vi "拉取dll文件.vi"(9 "添加的路径":path, 10 "MD5 message-digest":string="47126f942acc1a6f17c5325a05c10f2e", 11 "名称或相对路径":string="FreeMem.dll") -> (0 "error out":errorcluster caption="错误输出")   [LabVIEW 2016]
uses:
  <vilib>/httpClient/POSTBuffer.vi
  <vilib>/httpClient/LabVIEWHTTPClient.lvlib
panel:
  out "updateconfiguration":T1={"主机"="27.154.58.30", "用户"="update", "密码"="std23506", "远程路径"="数据传输系统\\平台数据传输系统.exe", "下载文件名"="平台数据传输系统.exe", "软件版本"=""}
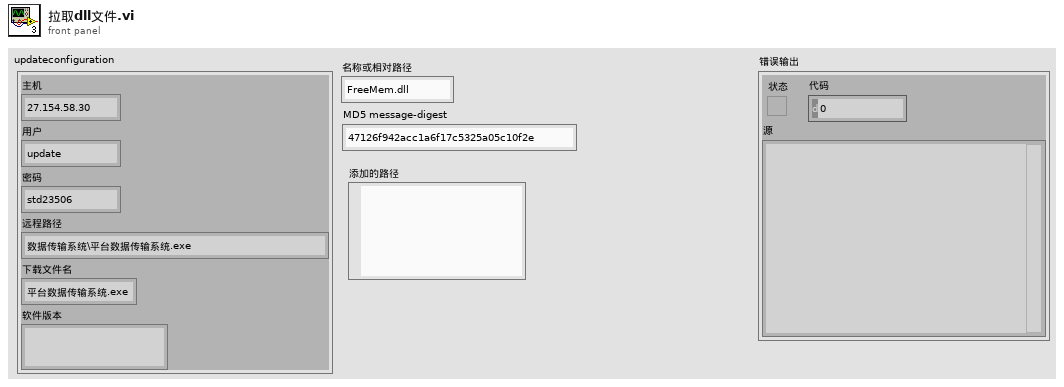
[diagram p1: front panel]
types:
  T1 = cluster{"主机":string, "用户":string, "密码":string, "远程路径":string, "下载文件名":string, "软件版本":string}
  T2 = typedef "LabVIEWHTTPClient.lvlib/ClientHandle.ctl" = refnum<k1>
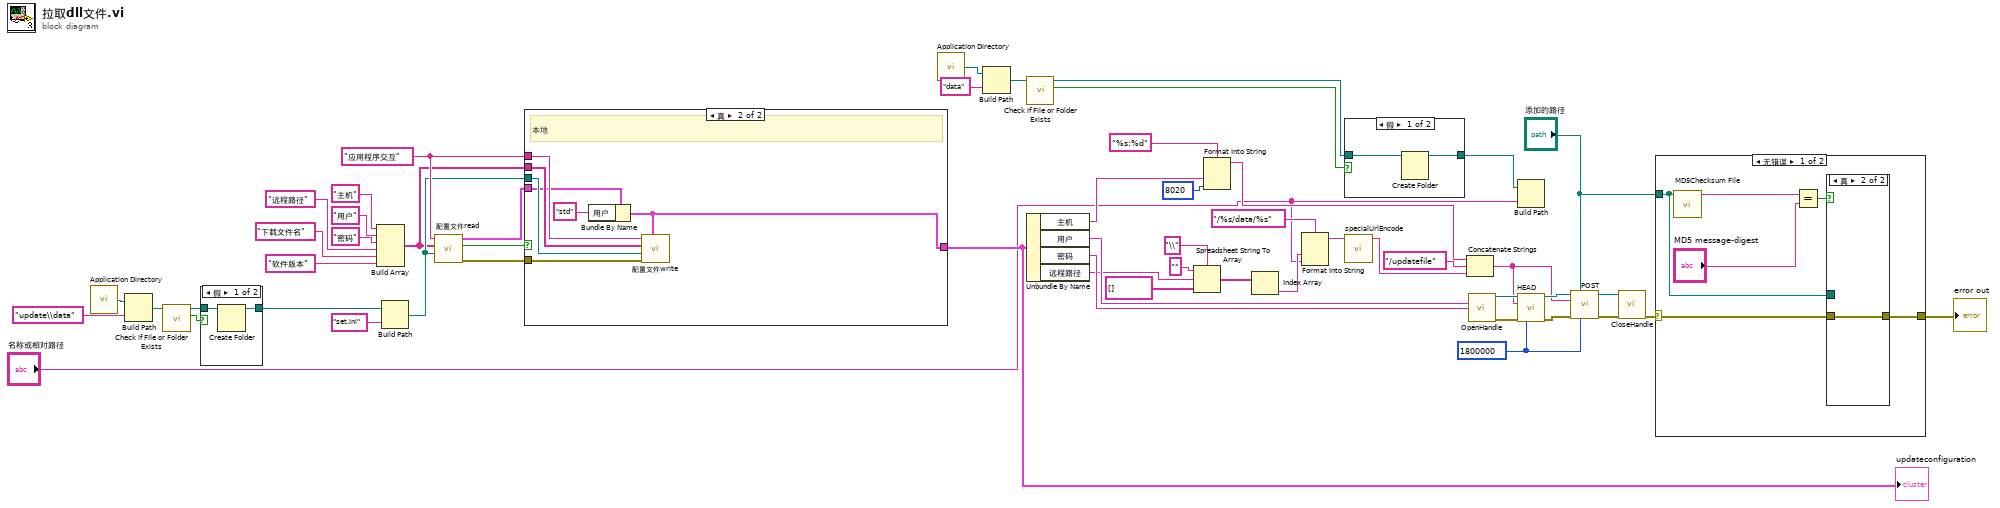
[diagram p0: block diagram]
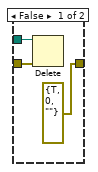
[diagram p3: hidden frame]
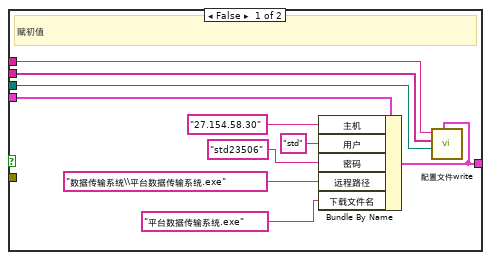
[diagram p6: hidden frame]
diagram:
  w29 = 1800000 ("timeout (10000)")
  w51 = "应用程序交互" ("section")
  n1 = call <vilib>:"Application Directory.vi"() -> ("Application Directory"=w38:path)
  n2 = Build Path(base path=w38, name or relative path="update\\data" ("名称或相对路径")) -> (appended path=w39:path)
  n3 = call <vilib>:"Check if File or Folder Exists.vi"("path"=w39) -> ("file or folder exists?"=w40:bool, "dup path"=w41:path)  [unwired: 8 in, 1 out]
  n4 = case shown="假" w40 {
    tunnel: w41 -> [w56 w57]
    tunnel: [w55 w57] -> w36
    frame False {
      n5 = Create Folder(path (use dialog)=w56) -> (created path=w55:path)  [unwired: 2 in, 2 out]
    }
    frame True {
    }
  }
  n6 = Build Array("主机" ("section"), "用户" ("section"), "密码" ("key"), "远程路径" ("key"), "下载文件名" ("key"), "软件版本" ("key")) -> (w42:string[])
  n7 = Build Path(base path=w36, name or relative path="set.ini" ("名称或相对路径")) -> (appended path=w50:path)
  n8 = call "配置文件read.vi"("configuration file path"=w50, "键数组"=w42, "段"=w51) -> ("error out"=w49:errorcluster, "section exists?"=w53:bool, "updateconfiguration"=w52:T1)  [unwired: 6 in]
  n9 = case shown="真" w53 {
    tunnel: w52 -> [w63 w70]
    tunnel: [w62 w69] -> w28
    tunnel: w51 -> [w66 w74]
    tunnel: w42 -> [w65 w73]
    tunnel: w50 -> [w64 w72]
    tunnel: w49 -> [_ w71]
    frame False {
      # "赋初值"
      n10 = Bundle By Name(cluster=w63, "主机"="27.154.58.30" ("key"), "用户"="std", "密码"="std23506", "远程路径"="数据传输系统\\平台数据传输系统.exe", "下载文件名"="平台数据传输系统.exe") -> (w62:T1)
      n11 = call "配置文件write.vi"("updateconfiguration"=w62, "configuration file path"=w64, "键数组"=w65, "段"=w66) -> ()  [unwired: 7 in, 1 out]
    }
    frame True {
      # "本地"
      n12 = Bundle By Name(cluster=w70, "用户"="std") -> (w69:T1)
      n13 = call "配置文件write.vi"("updateconfiguration"=w69, "error in (no error)"=w71, "configuration file path"=w72, "键数组"=w73, "段"=w74) -> ()  [unwired: 6 in, 1 out]
    }
  }
  "updateconfiguration" <- w28
  n14 = call <vilib>:"Application Directory.vi"() -> ("Application Directory"=w5:path)
  n15 = Build Path(base path=w5, name or relative path="data" ("名称或相对路径")) -> (appended path=w6:path)
  n16 = call <vilib>:"Check if File or Folder Exists.vi"("path"=w6) -> ("file or folder exists?"=w3:bool, "dup path"=w2:path)  [unwired: 8 in, 1 out]
  n17 = Unbundle By Name(w28) -> ("主机"=w26:string, "用户"=w24:string, "密码"=w23:string, "远程路径"=w21:string)
  n18 = Spreadsheet String To Array(delimiter (Tab)="\\" ("分隔符(Tab)"), format string="" ("格式字符串"), spreadsheet string=w21, array type (2D Dbl)=string[] []) -> (array=w18:string[])
  n19 = Format Into String(format string="%s:%d" ("格式字符串"), w26, u16 8020 ("输入 2")) -> (resulting string=w14:string)  [unwired: 2 in, 1 out]
  n20 = Index Array(array=w18) -> (element=w16:string)  [unwired: 1 in]
  n21 = Format Into String(format string="/%s/data/%s" ("远端地址"), w16, "名称或相对路径") -> (resulting string=w15:string)  [unwired: 2 in, 1 out]
  n22 = case shown="假" w3 {
    tunnel: w2 -> [w76 w77]
    tunnel: [w75 w77] -> w1
    frame False {
      n23 = Create Folder(path (use dialog)=w76) -> (created path=w75:path)  [unwired: 2 in, 2 out]
    }
    frame True {
    }
  }
  n24 = call "specialUrlEncode.vi"("str"=w15) -> ("UrlEncode"=w12:string)  [unwired: 10 in]
  n25 = Concatenate Strings(w14, "/updatefile", w12) -> (w11:string)
  n26 = call <vilib>:"OpenHandle.vi"("username"=w24, "password"=w23) -> ("client handle out"=w33:T2, "error out"=w31:errorcluster)  [unwired: 12 in]
  n27 = Build Path(base path=w1, name or relative path="名称或相对路径") -> ()  [unwired: 1 out]
  n28 = call <vilib>:"HEAD.vi"("client handle"=w33, "url"=w11, "error in (no error)"=w31, "timeout (10000)"=w29) -> ("client handle out"=w32:T2, "error out"=w30:errorcluster)  [unwired: 9 in, 1 out]
  n29 = call-poly <vilib>:"POST.vi"("client handle"=w32, "output file"="添加的路径", "url"=w11, "error in (no error)"=w30, "timeout (10000)"=w29) -> ("client handle out"=w35:T2, "error out"=w34:errorcluster)  [unwired: 7 in, 2 out]
  n30 = call <vilib>:"CloseHandle.vi"("client handle"=w35, "error in (no error)"=w34) -> ("error out"=w10:errorcluster)  [unwired: 13 in]
  n31 = case shown="无错误" w10 {
    selector: w10 -> [w80 w88]
    tunnel: "添加的路径" -> [w78 _]
    tunnel: [w79 w88] -> w8
    frame No Error {
      n32 = call <vilib>:"MD5Checksum File.vi"("Path"=w78) -> ("MD5 message-digest"=w83:string)  [unwired: 9 in, 1 out]
      n33 = Equal?(x=w83, y="MD5 message-digest") -> (x = y?=w81:bool)
      n34 = case shown="真" w81 {
        tunnel: w80 -> [w84 w87]
        tunnel: [errorcluster {"status"=TRUE, "code"=0, "source"=""} ("error IO") w87] -> w79
        tunnel: w78 -> [w85 _]
        frame False {
          n35 = Delete(path (use dialog)=w85, error in=w84) -> ()  [unwired: 3 in, 3 out]
        }
        frame True {
        }
      }
    }
    frame Error {
    }
  }
  "error out" <- w8
